vi "Enqueue-Command.vi"(6 "Timeout [ms] (-1)":i32=-1, 7 "Has Priority (F)":bool, 8 "error in (no error)":errorcluster, 9 "Cmd Data":variant, 10 "Cmd":T1, 11 "Engine in":refnum<class "Engine.lvclass">) -> (0 "error out":errorcluster, 2 "Timeout?":bool, 3 "Engine out":refnum<class "Engine.lvclass">)   [LabVIEW 2024, in "GLF.lvlib" / "Engine.lvclass"]
uses:
  Engine.lvclass
  Engine.lvclass/Engine.ctl
  Command--enum.ctl
  Command--cluster.ctl
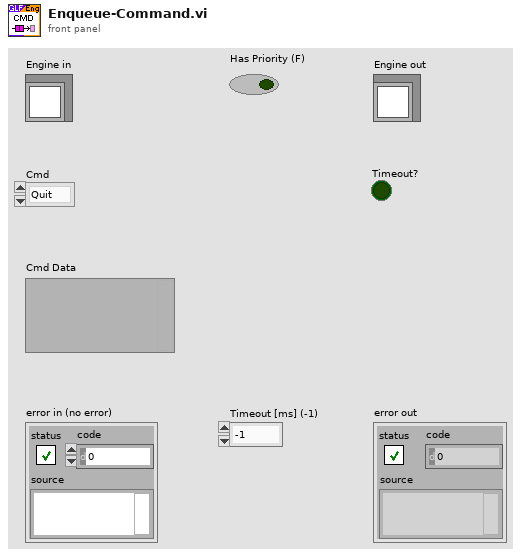
[diagram p1: front panel]
types:
  T1 = typedef "GLF.lvlib/Engine.lvclass/Command--enum.ctl" = enum16{"Quit", "Register Window"}
  T2 = typedef "GLF.lvlib/Engine.lvclass/Command--cluster.ctl" = cluster{"Cmd":T1, "Data":variant}
  T3 = typedef "GLF.lvlib/Engine.lvclass/DVR--cluster.ctl" = cluster{"CMD Queue":T4, "Config":T5, "Ctxt":T7, "Metrics":T8, "GLF Instances":set{refnum<class "IAmGLF.lvclass">}, "Window Instances":map{i64, refnum<class "Window.lvclass">}}
  T4 = typedef "GLF.lvlib/Engine.lvclass/Command--queue.ctl" = refnum<queue>
  T5 = typedef "GLF.lvlib/Engine.lvclass/Config--cluster.ctl" = cluster{"Quit On Last Window Closed":bool, "VSync":T6, "FPS Target":dbl}
  T6 = typedef "GLF.lvlib/Engine.lvclass/VSync--enum.ctl" = enum16{"Disabled", "Enabled", "Adaptative"}
  T7 = typedef "GLF.lvlib/Engine.lvclass/Context--cluster.ctl" = cluster{"Ticks Begin":u64, "VSync Enabled":bool}
  T8 = typedef "GLF.lvlib/Engine.lvclass/Metrics--cluster.ctl" = cluster{"Uptime [ms]":u64, "Loop Time [ms]":u64}
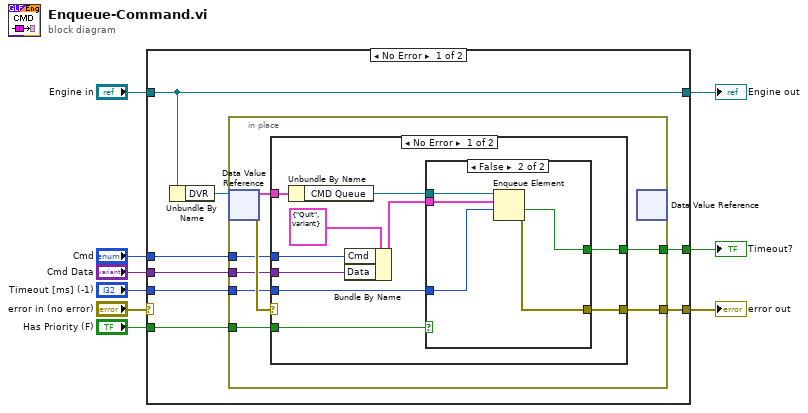
[diagram p0: block diagram]
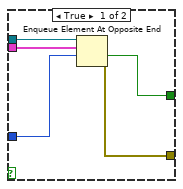
[diagram p2: hidden frame]
diagram:
  n1 = case shown="No Error" "error in (no error)" {
    selector: "error in (no error)" -> [_ w48]
    tunnel: "Engine in" -> [w11 w47]
    tunnel: [w17 w48] -> w8
    tunnel: "Cmd" -> [w16 _]
    tunnel: "Cmd Data" -> [w15 _]
    tunnel: "Timeout [ms] (-1)" -> [w14 _]
    tunnel: [w13 _] -> w4
    tunnel: "Has Priority (F)" -> [w12 _]
    tunnel: [w11 w47] -> w1
    frame No Error {
      n2 = Unbundle By Name(w11) -> ("DVR"=w10:refnum<data-value>)
      n3 = in-place {
        in-place-border: [w24] -> w17
        in-place-border: w16 -> [w23]
        in-place-border: w15 -> [w22]
        in-place-border: w14 -> [w21]
        in-place-border: [w20] -> w13
        in-place-border: w12 -> [w19]
        n4 = in-place-dvr #1(w10) -> (w18:T3, w25:errorcluster)
        n5 = case shown="No Error" w25 {
          selector: w25 -> [_ w46]
          tunnel: [w35 w46] -> w24
          tunnel: w23 -> [w32 _]
          tunnel: w22 -> [w31 _]
          tunnel: w21 -> [w30 _]
          tunnel: [w29 _] -> w20
          tunnel: w19 -> [w28 _]
          tunnel: w18 -> [w27 _]
          frame No Error {
            n6 = Unbundle By Name(w27) -> ("CMD Queue"=w26:T4)
            n7 = Bundle By Name(cluster=T2 {"Cmd"=enum."Quit", "Data"=variant} ("element"), "Cmd"=w32, "Data"=w31) -> (w33:T2)
            n8 = case shown="False" w28 {
              tunnel: w26 -> [w40 w45]
              tunnel: [w39 w44] -> w35
              tunnel: w33 -> [w38 w43]
              tunnel: w30 -> [w37 w42]
              tunnel: [w36 w41] -> w29
              frame True {
                n9 = Enqueue Element At Opposite End(queue=w40, element=w38, timeout in ms (-1)=w37) -> (timed out?=w36:bool, error out=w39:errorcluster)  [unwired: 1 in, 1 out]
              }
              frame False {
                n10 = Enqueue Element(queue=w45, element=w43, timeout in ms (-1)=w42) -> (timed out?=w41:bool, error out=w44:errorcluster)  [unwired: 1 in, 1 out]
              }
            }
          }
          frame Error {
          }
        }
        n11 = in-place-dvr #1() -> ()  [unwired: 1 in, 2 out]
      }
    }
    frame Error {
    }
  }
  "error out" <- w8
  "Engine out" <- w1
  "Timeout?" <- w4
